vi "parseReportServerStatusResponse.vi"(8 "error in (no error)":errorcluster, 10 "DynamicFrameParser":refnum<class "DynamicFrameParser.lvclass">, 11 "ILC in":refnum<class "ILC.lvclass">) -> (0 "error out":errorcluster, 3 "ILC out":refnum<class "ILC.lvclass">)   [LabVIEW 2016, in "RTILC.lvlib" / "ILC.lvclass"]
uses:
  ILC.lvclass
  Common_RT_Modbus/DynamicFrameParser/DynamicFrameParser.lvclass
  Common_RT_Modbus/DataTypes/ExceptionCodes.ctl
  ILC.lvclass/ILC.ctl
  Common_RT_Modbus/RTModbus.lvlib
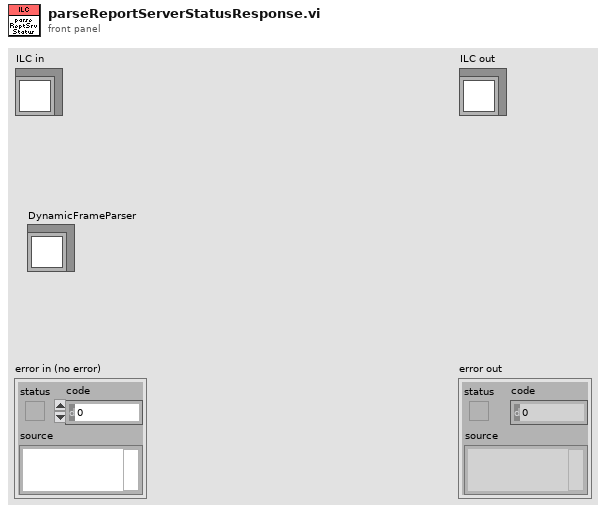
[diagram p1: front panel]
types:
  T1 = typedef "RTModbus.lvlib/ExceptionCodes.ctl" = u16
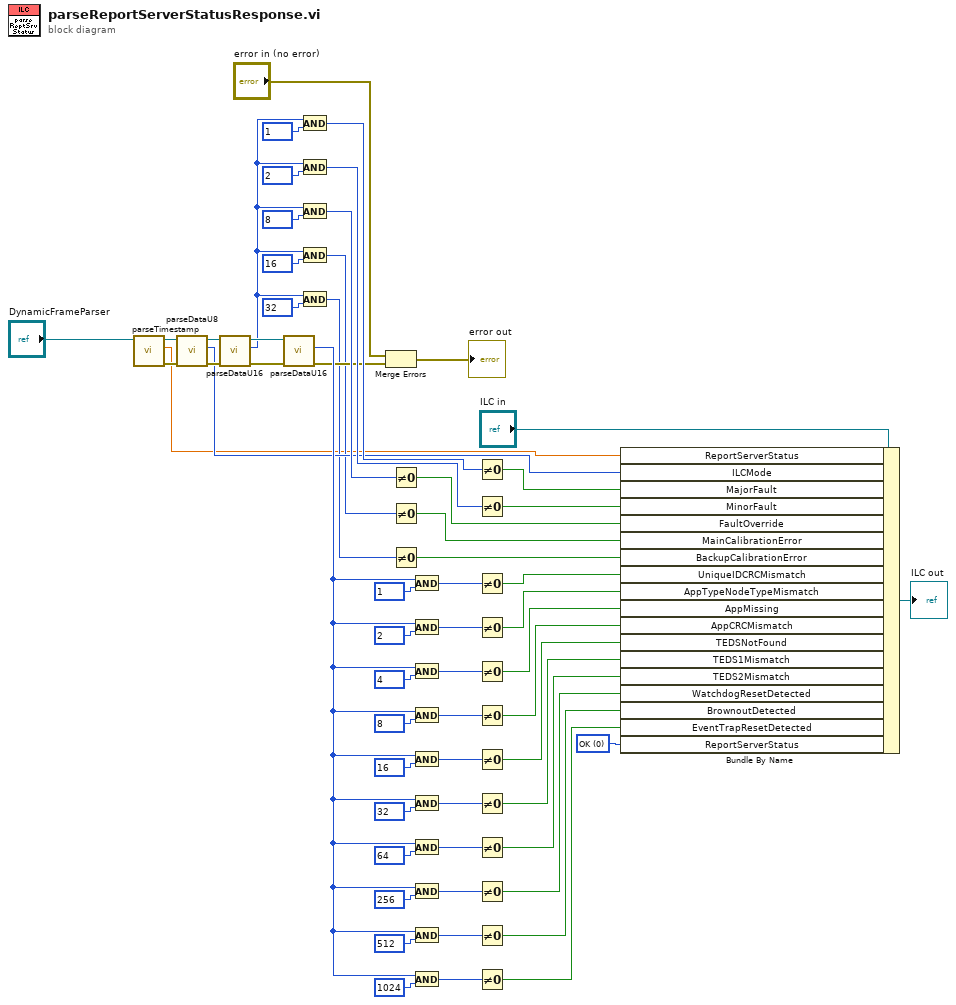
[diagram p0: block diagram]
diagram:
  w12 = T1 0 items=["OK", "IllegalFunction", "IllegalDataAddress", "IllegalDataValue", "SlaveDeviceFailure", "Acknowledge", "SlaveDeviceBusy", "NegativeAcknowledge", "MemoryParityError", "GatewayPathUnavailable", "GatewayTargetDeviceFailedToRespond"] ("ILCData.Responses.ReportServerStatus")
  n1 = call "parseTimestamp.vi"("FrameParser in"="DynamicFrameParser") -> ("error out"=w2:errorcluster, "Timestamp"=w1:dbl, "FrameParser out"=w3:refnum<class "DynamicFrameParser.lvclass">)  [unwired: 8 in]
  n2 = call "parseDataU8.vi"("error in (no error)"=w2, "FrameParser in"=w3) -> ("error out"=w20:errorcluster, "Data"=w18:u8, "FrameParser out"=w19:refnum<class "DynamicFrameParser.lvclass">)  [unwired: 7 in]
  n3 = call "parseDataU16.vi"("error in (no error)"=w20, "FrameParser in"=w19) -> ("error out"=w30:errorcluster, "Data"=w11:u16, "FrameParser out"=w31:refnum<class "DynamicFrameParser.lvclass">)  [unwired: 7 in]
  n4 = call "parseDataU16.vi"("error in (no error)"=w30, "FrameParser in"=w31) -> ("error out"=w17:errorcluster, "Data"=w32:u16)  [unwired: 7 in, 1 out]
  n5 = And(x=w11, y=u16 1) -> (x .and. y?=w24:u16)
  n6 = And(x=w11, y=u16 2) -> (x .and. y?=w25:u16)
  n7 = And(x=w11, y=u16 8) -> (x .and. y?=w26:u16)
  n8 = And(x=w11, y=u16 16) -> (x .and. y?=w8:u16)
  n9 = And(x=w11, y=u16 32) -> (x .and. y?=w7:u16)
  n10 = Merge Errors("error in (no error)", w17) -> (→"error out":errorcluster)
  n11 = Not Equal To 0?(x=w26) -> (x != 0?=w29:bool)
  n12 = Not Equal To 0?(x=w8) -> (x != 0?=w6:bool)
  n13 = Not Equal To 0?(x=w7) -> (x != 0?=w5:bool)
  n14 = And(x=w32, y=u16 1) -> (x .and. y?=w42:u16)
  n15 = And(x=w32, y=u16 2) -> (x .and. y?=w41:u16)
  n16 = And(x=w32, y=u16 4) -> (x .and. y?=w40:u16)
  n17 = And(x=w32, y=u16 8) -> (x .and. y?=w39:u16)
  n18 = And(x=w32, y=u16 16) -> (x .and. y?=w38:u16)
  n19 = And(x=w32, y=u16 32) -> (x .and. y?=w37:u16)
  n20 = And(x=w32, y=u16 64) -> (x .and. y?=w36:u16)
  n21 = And(x=w32, y=u16 256) -> (x .and. y?=w35:u16)
  n22 = And(x=w32, y=u16 512) -> (x .and. y?=w34:u16)
  n23 = And(x=w32, y=u16 1024) -> (x .and. y?=w33:u16)
  n24 = Not Equal To 0?(x=w24) -> (x != 0?=w27:bool)
  n25 = Not Equal To 0?(x=w25) -> (x != 0?=w28:bool)
  n26 = Not Equal To 0?(x=w42) -> (x != 0?=w53:bool)
  n27 = Not Equal To 0?(x=w41) -> (x != 0?=w54:bool)
  n28 = Not Equal To 0?(x=w40) -> (x != 0?=w55:bool)
  n29 = Not Equal To 0?(x=w39) -> (x != 0?=w56:bool)
  n30 = Not Equal To 0?(x=w38) -> (x != 0?=w57:bool)
  n31 = Not Equal To 0?(x=w37) -> (x != 0?=w58:bool)
  n32 = Not Equal To 0?(x=w36) -> (x != 0?=w59:bool)
  n33 = Not Equal To 0?(x=w35) -> (x != 0?=w60:bool)
  n34 = Not Equal To 0?(x=w34) -> (x != 0?=w61:bool)
  n35 = Not Equal To 0?(x=w33) -> (x != 0?=w62:bool)
  n36 = Bundle By Name(cluster="ILC in", "ReportServerStatus"=w1, "ILCMode"=w18, "MajorFault"=w27, "MinorFault"=w28, "FaultOverride"=w29, "MainCalibrationError"=w6, "BackupCalibrationError"=w5, "UniqueIDCRCMismatch"=w53, "AppTypeNodeTypeMismatch"=w54, "AppMissing"=w55, "AppCRCMismatch"=w56, "TEDSNotFound"=w57, "TEDS1Mismatch"=w58, "TEDS2Mismatch"=w59, "WatchdogResetDetected"=w60, "BrownoutDetected"=w61, "EventTrapResetDetected"=w62, "ReportServerStatus"=w12) -> (→"ILC out":refnum<class "ILC.lvclass">)
